vi "ParseXMLFragments.vi"(8 "error in (no error)":errorcluster, 10 "XML in":string) -> (0 "error out":errorcluster, 2 "XML Elements":string[](array[string]))   [LabVIEW 2020]
doc: "This VI parses its XML code input and returns an array of the top level elements."
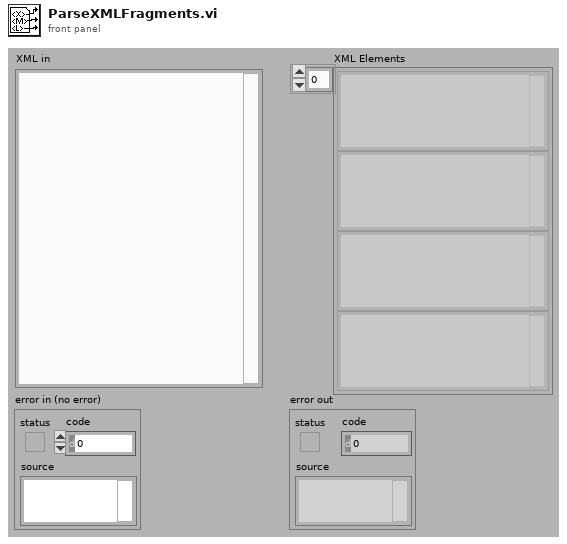
[diagram p1: front panel]
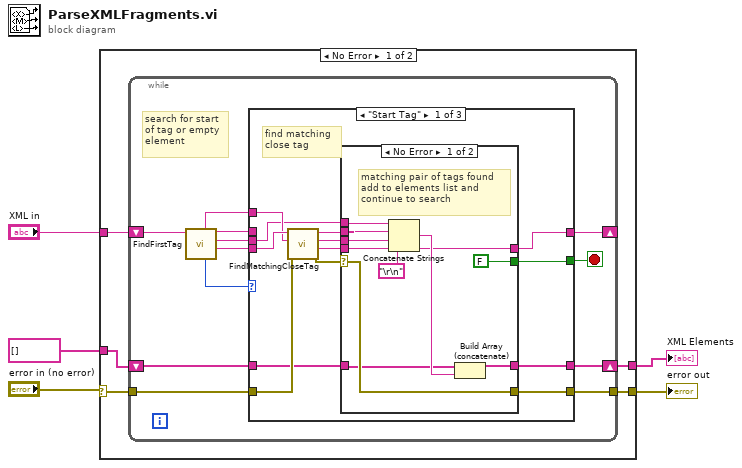
[diagram p0: block diagram]
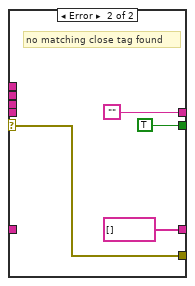
[diagram p2: hidden frame]
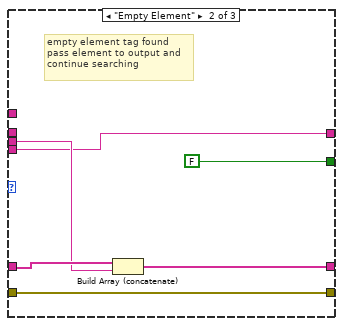
[diagram p3: hidden frame]
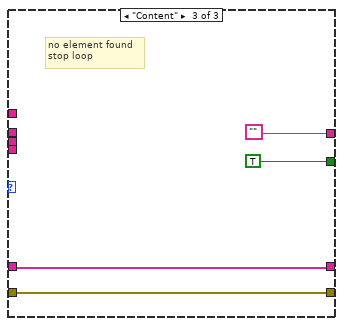
[diagram p4: hidden frame]
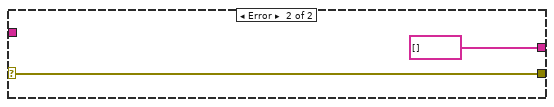
[diagram p5: hidden frame]
diagram:
  n1 = case shown="No Error" "error in (no error)" {
    selector: "error in (no error)" -> [w7 w61]
    tunnel: "XML in" -> [w10 _]
    tunnel: string[] [] -> [w9 _]
    tunnel: [w8 string[] []] -> w3
    tunnel: [w6 w61] -> w1
    frame No Error {
      n2 = while {
        shift-right: [w22] -> _
        shift-left: w10 -> [w16]
        shift-right: [w19] -> w8
        shift-left: w9 -> [w20]
        tunnel: w7 -> [w18]
        tunnel: [w17] -> w6
        stop <- w21 stop-if-true
        # "search for start\nof tag or empty\nelement"
        n3 = call "FindFirstTag.vi"("XML String In"=w16) -> ("after tag"=w11:string, "tag"=w12:string, "before tag"=w13:string, "case"=w15:enum16{"Start Tag", "Empty Element", "Content"}, "element name"=w14:string)  [unwired: 1 in, 5 out]
        n4 = case shown="\"Start Tag\"" w15 {
          tunnel: [w29 w51 ""] -> w22
          tunnel: [w23 FALSE TRUE] -> w21
          tunnel: w20 -> [w31 w55 w56]
          tunnel: [w27 w53 w56] -> w19
          tunnel: w18 -> [w33 w52 w59]
          tunnel: [w28 w52 w59] -> w17
          tunnel: w14 -> [w34 _ _]
          tunnel: w13 -> [_ _ _]
          tunnel: w12 -> [w30 w54 _]
          tunnel: w11 -> [w35 w51 _]
          frame "Start Tag" {
            # "find matching\nclose tag"
            n5 = call "FindMatchingCloseTag.vi"("error in"=w33, "element name"=w34, "XML string in"=w35) -> ("error out"=w32:errorcluster, "text after end tag"=w24:string, "close tag"=w25:string, "string before end tag"=w26:string)  [unwired: 5 out]
            n6 = case shown="No Error" w32 {
              selector: w32 -> [w43 w49]
              tunnel: w26 -> [w44 _]
              tunnel: w31 -> [w41 _]
              tunnel: w30 -> [w45 _]
              tunnel: [w38 ""] -> w29
              tunnel: [w43 w49] -> w28
              tunnel: [w40 string[] []] -> w27
              tunnel: w25 -> [w39 _]
              tunnel: w24 -> [w38 _]
              tunnel: [FALSE TRUE] -> w23
              frame No Error {
                # "matching pair of tags found\nadd to elements list and\ncontinue to search"
                n7 = Concatenate Strings(w45, w44, w39, "\r\n") -> (w42:string)
                n8 = Build Array (concatenate)(w41, w42) -> (w40:string[])
              }
              frame Error {
                # "no matching close tag found"
              }
            }
          }
          frame "Empty Element" {
            # "empty element tag found\npass element to output and\ncontinue searching"
            n9 = Build Array (concatenate)(w55, w54) -> (w53:string[])
          }
          frame "Content" {
            # "no element found\nstop loop"
          }
        }
      }
    }
    frame Error {
    }
  }
  "XML Elements" <- w3
  "error out" <- w1
